vi "cluster_v13.vi"() -> ()   [LabVIEW 2009]
panel:
  out "Afisare grafic X-logaritmic":cluster{dbl[], dbl[]}(graph)
  out "Afisare  grafic - x proportional":dbl[](graph)
  out "Array":dbl[](array[numeric])
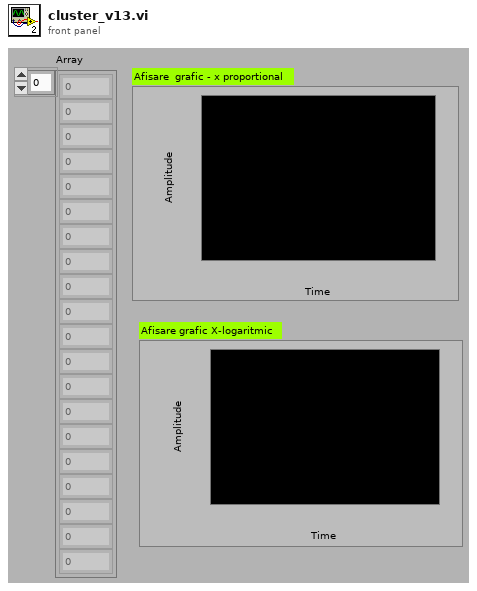
[diagram p1: front panel]
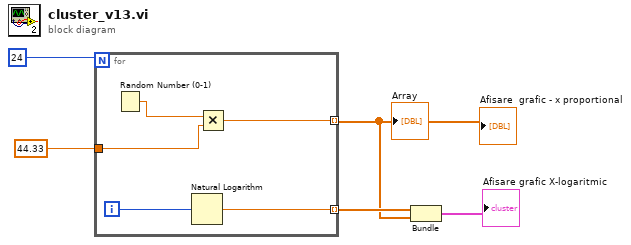
[diagram p0: block diagram]
diagram:
  n1 = for {
    N: 24 -> [_]
    tunnel: 44.33 -> [w9]
    tunnel: [w10] -> w1 mode=indexing
    tunnel: [w6] -> w2 mode=indexing
    i -> [w7]
    n2 = Random Number (0-1)() -> (number: 0 to 1=w8:dbl)
    n3 = Natural Logarithm(1:w7) -> (0:w6:dbl)
    n4 = Multiply(x=w8, y=w9) -> (x*y=w10:dbl)
  }
  "Array" <- w1
  "Afisare  grafic - x proportional" <- w1
  n5 = Bundle(w2, w1) -> (→"Afisare grafic X-logaritmic":cluster{dbl[], dbl[]})  [unwired: 1 in]
